vi "例程04-数组与簇.vi"() -> ()   [LabVIEW 2018]
panel:
  out "布尔 2":bool
  in  "布尔":bool
  in  "簇":cluster{"数值":dbl, "布尔":bool, "字符串":string}
  out "索引第一行第二列元素":dbl
  out "大小":i32[](array[numeric])
  in  "数组":dbl[][](array[numeric])
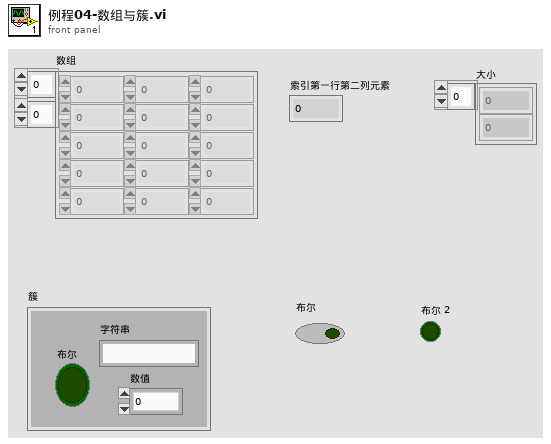
[diagram p1: front panel]
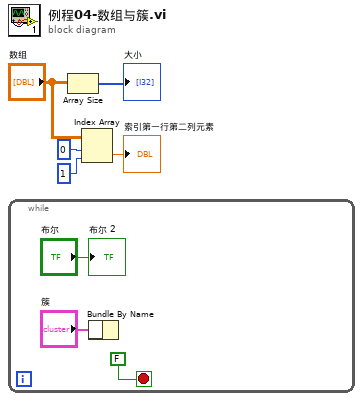
[diagram p0: block diagram]
diagram:
  n1 = while {
    stop <- FALSE stop-if-true
    n2 = Bundle By Name("簇") -> ()  [unwired: 1 in, 1 out]
    "布尔 2" <- "布尔"
  }
  n3 = Array Size(array="数组") -> (size(s)=→"大小":i32[])
  n4 = Index Array(array="数组", index (row)=0 ("索引 (行)"), index (col)=1 ("禁用的索引 (列)")) -> (element=→"索引第一行第二列元素":dbl)
